vi "FTW-PerfTest-JSON-Fetch.vi"() -> (0 "Test Result":errorcluster)   [LabVIEW 2015]
uses:
  src/json/core/FTW-JSON-Core-Type.ctl
  src/reflection/FTW-Reflection-Types.ctl
  src/time/FTW-Time-RelativeTimer.vi
  lib/FTW-KernelFilepath.vi
  src/json/core/FTW-JSON-Core-NumericType.vi
  src/error/FTW-ERR-ThrowError.vi
  src/error/FTW-ERR-ThrowInvalidReferenceError.vi
  src/json/core/FTW-JSON-Core-ElementType.vi
  codegen/xnode/FTW-Dataflow-Synchronizer.xnode
  codegen/xnode/FTW-JSON-Fetch.xnode
  src/json/FTW-JSON-Type.ctl
panel:
  out "Waveform Chart":T1(graph)
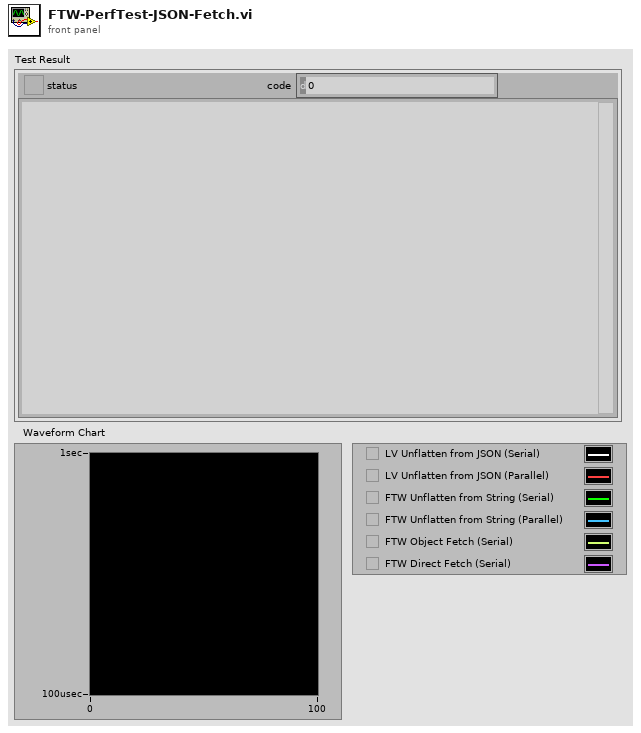
[diagram p1: front panel]
types:
  T1 = cluster{"[0]":dbl, "[1]":dbl, "[2]":dbl, "[3]":dbl, "[4]":dbl, "[5]":dbl}
  T2 = enum16{"LV Unflatten from JSON (Serial)", "LV Unflatten from JSON (Parallel)", "FTW Unflatten from String (Serial)", "FTW Unflatten from String (Parallel)", "FTW Object Fetch (Serial)", "FTW Direct Fetch (Serial)"}
  T3 = typedef "FTW-Type-JSON.ctl" = refnum<data-value>
  T4 = typedef "FTW-JSON-Core-Type.ctl" = enum8{"Object", "Array", "String", "Integer", "Floating Point", "true", "false", "null", "undefined"}
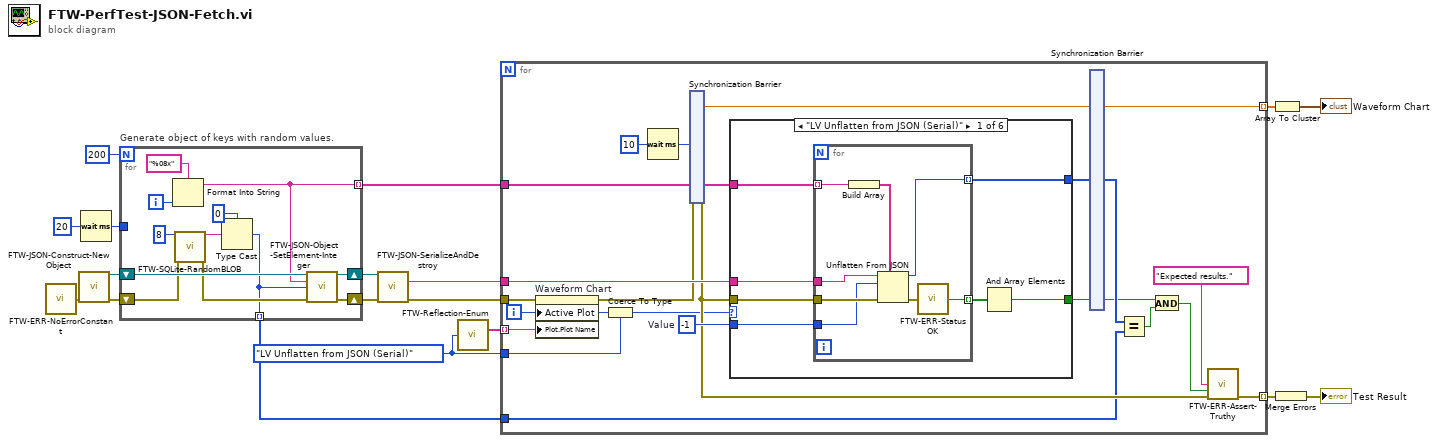
[diagram p0: block diagram]
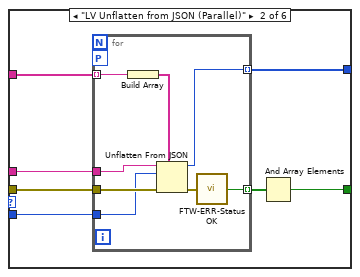
[diagram p2: hidden frame]
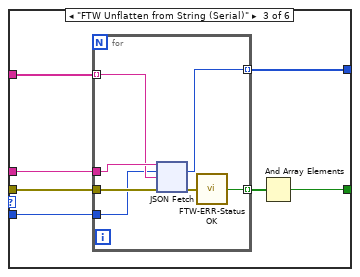
[diagram p3: hidden frame]
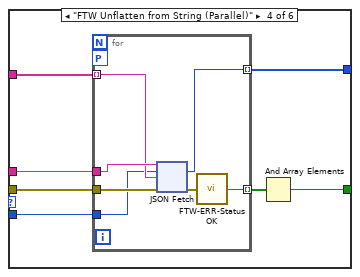
[diagram p4: hidden frame]
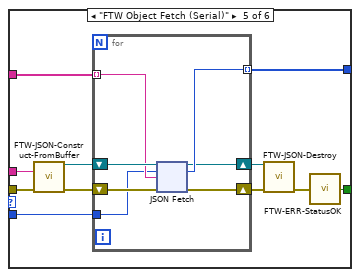
[diagram p5: hidden frame]
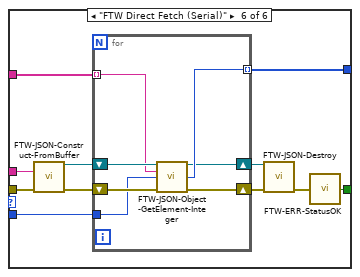
[diagram p6: hidden frame]
diagram:
  w3 = T2."LV Unflatten from JSON (Serial)"
  n1 = call "FTW-ERR-NoErrorConstant.vi"() -> ("no error"=w18:errorcluster)
  n2 = call "FTW-JSON-Construct-NewObject.vi"("error in"=w18) -> ("JSON"=w17:T3, "error out"=w16:errorcluster)  [unwired: 13 in]
  n3 = Wait (ms)(milliseconds to wait=u32 20) -> (millisecond timer value=w1:u32)
  n4 = for "Generate object of keys with random values." {
    N: 200 -> [_]
    shift-right: [w26] -> w14
    shift-left: w16 -> [w23]
    shift-right: [w29] -> w11
    shift-left: w17 -> [w30]
    tunnel: [w19] -> w10 mode=indexing
    tunnel: [w25] -> w12 mode=indexing
    tunnel: w1 -> [_]
    i -> [w28]
    n5 = Format Into String(format string="%08x", w28) -> (resulting string=w25:string)  [unwired: 2 in, 1 out]
    n6 = call "FTW-SQLite-RandomBLOB.vi"("Number of Bytes"=8, "error in"=w23) -> ("Random BLOB"=w21:string, "error out"=w22:errorcluster)  [unwired: 12 in]
    n7 = Type Cast(type=i64 0 ("64bit integer"), x=w21) -> (*(type *) &x=w19:i64)
    n8 = call "FTW-JSON-Object-SetElement-Integer.vi"("JSON"=w30, "Key"=w25, "Value"=w19, "error in"=w22) -> ("JSON out"=w29:T3, "error out"=w26:errorcluster)  [unwired: 10 in]
  }
  n9 = call "FTW-JSON-SerializeAndDestroy.vi"("JSON"=w11, "error in"=w14) -> ("JSON String (UTF-8)"=w13:string, "error out"=w9:errorcluster)  [unwired: 12 in]
  n10 = call "FTW-Reflection-Enum.vi"("Enum"=w3) -> ("Enum Items"=w4:string[])  [unwired: 12 in, 2 out]
  n11 = for {
    tunnel: [w48] -> w6 mode=indexing
    tunnel: w13 -> [w54]
    tunnel: w12 -> [w51]
    tunnel: w10 -> [w31]
    tunnel: w4 -> [w38] mode=indexing
    tunnel: w9 -> [w37]
    tunnel: [w40] -> w8 mode=indexing
    tunnel: w3 -> [w35]
    i -> [w32]
    w46 = i64 -1  # Value
    n12 = property on="Waveform Chart" class="WFChart (strict)"(error in=w37, "Active Plot"=w32, "Plot.Plot Name"=w38) -> (error out=w33:errorcluster)  [unwired: 1 in, 1 out]
    n13 = Coerce To Type(0:w32, 1:w35) -> (2:w34:T2)
    n14 = Wait (ms)(milliseconds to wait=u32 10) -> (millisecond timer value=w52:u32)
    n15 = xnode "Synchronization Barrier"("Synchronized Signal 1"=w52, "Synchronized Signal 2"=w51, w33) -> ("High-Resolution Timer"=w49:dbl, "out"=w50:string[], "error IO out"=w36:errorcluster)  [unwired: 5 in, 2 out]
    n16 = case shown="\"LV Unflatten from JSON (Serial)\"" w34 {
      tunnel: w54 -> [w61 w76 w91 w161 w232 w302]
      tunnel: w50 -> [w60 w75 w90 w160 w235 w305]
      tunnel: [w56 w71 w85 w155 w225 w295] -> w47
      tunnel: w36 -> [w59 w74 w89 w159 w231 w301]
      tunnel: w46 -> [w58 w73 w88 w158 w234 w304]
      tunnel: [w57 w72 w87 w157 w233 w303] -> w45
      frame "LV Unflatten from JSON (Serial)" {
        n17 = for {
          tunnel: w61 -> [w68]
          tunnel: w59 -> [w69]
          tunnel: w60 -> [w65] mode=indexing
          tunnel: w58 -> [w66]
          tunnel: [w63] -> w57 mode=indexing
          tunnel: [w62] -> w55 mode=indexing
          n18 = Build Array(w65) -> (w64:string[])
          n19 = Unflatten From JSON(path=w64, JSON string=w68, type and defaults=w66, error in (no error)=w69) -> (value=w63:i64, error out=w67:errorcluster)  [unwired: 3 in]
          n20 = call "FTW-ERR-StatusOK.vi"("error to check"=w67) -> ("Status OK?"=w62:bool)
        }
        n21 = And Array Elements(Boolean array=w55) -> (logical AND=w56:bool)
      }
      frame "LV Unflatten from JSON (Parallel)" {
        n22 = for {
          workers-P: _ -> [_]
          tunnel: w76 -> [w83]
          tunnel: w74 -> [w84]
          tunnel: w75 -> [w80] mode=indexing
          tunnel: w73 -> [w81]
          tunnel: [w78] -> w72 mode=indexing
          tunnel: [w77] -> w70 mode=indexing
          n23 = Build Array(w80) -> (w79:string[])
          n24 = Unflatten From JSON(path=w79, JSON string=w83, type and defaults=w81, error in (no error)=w84) -> (value=w78:i64, error out=w82:errorcluster)  [unwired: 3 in]
          n25 = call "FTW-ERR-StatusOK.vi"("error to check"=w82) -> ("Status OK?"=w77:bool)
        }
        n26 = And Array Elements(Boolean array=w70) -> (logical AND=w71:bool)
      }
      frame "FTW Unflatten from String (Serial)" {
        n27 = for {
          tunnel: w91 -> [w97]
          tunnel: w89 -> [w98]
          tunnel: w90 -> [w96] mode=indexing
          tunnel: w88 -> [w95]
          tunnel: [w94] -> w87 mode=indexing
          tunnel: [w92] -> w86 mode=indexing
          n28 = xnode "JSON Fetch"("JSON"=w97, "Element Type and Default Value"=w95, "Element Path"=w96, "error in"=w98) -> ("Value"=w94:i64, "error out"=w93:errorcluster)  [unwired: 1 in, 3 out]
          n29 = call "FTW-ERR-StatusOK.vi"("error to check"=w93) -> ("Status OK?"=w92:bool)
        }
        n30 = And Array Elements(Boolean array=w86) -> (logical AND=w85:bool)
      }
      frame "FTW Unflatten from String (Parallel)" {
        n31 = for {
          workers-P: _ -> [_]
          tunnel: w161 -> [w167]
          tunnel: w159 -> [w168]
          tunnel: w160 -> [w166] mode=indexing
          tunnel: w158 -> [w165]
          tunnel: [w164] -> w157 mode=indexing
          tunnel: [w162] -> w156 mode=indexing
          n32 = xnode "JSON Fetch"("JSON"=w167, "Element Type and Default Value"=w165, "Element Path"=w166, "error in"=w168) -> ("Value"=w164:i64, "error out"=w163:errorcluster)  [unwired: 1 in, 3 out]
          n33 = call "FTW-ERR-StatusOK.vi"("error to check"=w163) -> ("Status OK?"=w162:bool)
        }
        n34 = And Array Elements(Boolean array=w156) -> (logical AND=w155:bool)
      }
      frame "FTW Object Fetch (Serial)" {
        n35 = call "FTW-JSON-Construct-FromBuffer.vi"("JSON String (UTF-8)"=w232, "error in"=w231) -> ("JSON"=w229:T3, "error out"=w230:errorcluster)  [unwired: 12 in]
        n36 = for {
          tunnel: w235 -> [w240] mode=indexing
          tunnel: w234 -> [w239]
          tunnel: [w238] -> w233 mode=indexing
          shift-right: [w237] -> w228
          shift-left: w229 -> [w241]
          shift-right: [w236] -> w227
          shift-left: w230 -> [w242]
          n37 = xnode "JSON Fetch"("JSON"=w241, "Element Type and Default Value"=w239, "Element Path"=w240, "error in"=w242) -> ("JSON out"=w237:T3, "Value"=w238:i64, "error out"=w236:errorcluster)  [unwired: 1 in, 2 out]
        }
        n38 = call "FTW-JSON-Destroy.vi"("JSON"=w228, "error in"=w227) -> ("error out"=w226:errorcluster)  [unwired: 13 in]
        n39 = call "FTW-ERR-StatusOK.vi"("error to check"=w226) -> ("Status OK?"=w225:bool)
      }
      frame "FTW Direct Fetch (Serial)" {
        n40 = call "FTW-JSON-Construct-FromBuffer.vi"("JSON String (UTF-8)"=w302, "error in"=w301) -> ("JSON"=w299:T3, "error out"=w300:errorcluster)  [unwired: 12 in]
        n41 = for {
          tunnel: w305 -> [w310] mode=indexing
          tunnel: w304 -> [w309]
          tunnel: [w308] -> w303 mode=indexing
          shift-right: [w307] -> w298
          shift-left: w299 -> [w312]
          shift-right: [w306] -> w297
          shift-left: w300 -> [w311]
          n42 = call "FTW-JSON-Object-GetElement-Integer.vi"("JSON"=w312, "Key"=w310, "Default Value"=w309, "error in"=w311) -> ("JSON out"=w307:T3, "Value"=w308:i64, "error out"=w306:errorcluster)  [unwired: 8 in, 1 out]
        }
        n43 = call "FTW-JSON-Destroy.vi"("JSON"=w298, "error in"=w297) -> ("error out"=w296:errorcluster)  [unwired: 13 in]
        n44 = call "FTW-ERR-StatusOK.vi"("error to check"=w296) -> ("Status OK?"=w295:bool)
      }
    }
    n45 = xnode "Synchronization Barrier"("Upstream Timer Value"=w49, w45, "Synchronized Signal 1"=w47) -> ("Elapsed Time"=w48:dbl, "out"=w44:i64[], "error IO out"=w39:bool)  [unwired: 21 in, 1 out]
    n46 = Equal?(x=w44, y=w31) -> (x = y?=w43:bool)
    n47 = And(x=w39, y=w43) -> (x .and. y?=w42:bool)
    n48 = call "FTW-ERR-Assert-Truthy.vi"("Assertion"="Expected results.", "Assertion holds true?"=w42, "error in"=w36) -> ("error out"=w40:errorcluster)  [unwired: 12 in]
  }
  n49 = Array To Cluster(array=w6) -> (cluster=→"Waveform Chart":T1)
  n50 = Merge Errors(w8) -> (→"Test Result":errorcluster)
